vi "Pass Allowed Message.vi"(2 "Allowed Message":string[](array[string]), 3 "JKISM External Event":string) -> (1 "States":string)   [LabVIEW 2017, in "_jkism_magic.lvlib"]
uses:
  _jkism_magic.lvlib
  Communicable State Machine.lvlib
  _Shared/CSM Shared.lvlib
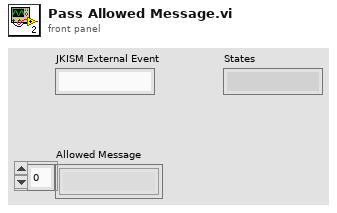
[diagram p1: front panel]
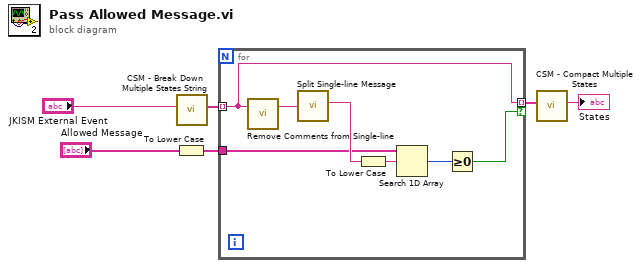
[diagram p0: block diagram]
diagram:
  n1 = To Lower Case(string="Allowed Message") -> (all lower case string=w3:string[])
  n2 = call "CSM - Break Down Multiple States String.vi"("States"="JKISM External Event") -> ("Multiple States"=w1:string[])  [unwired: 10 in]
  n3 = for {
    tunnel: w1 -> [w7] mode=indexing
    tunnel: [w7] -> w4 mode=indexing if=w8
    tunnel: w3 -> [w11]
    n4 = call "Remove Comments from Single-line.vi"("single-line text"=w7) -> ("single-line text without comments"=w13:string)  [unwired: 2 in]
    n5 = call "Split Single-line Message.vi"("single-line text"=w13) -> ("state"=w12:string)  [unwired: 6 in, 3 out]
    n6 = To Lower Case(string=w12) -> (all lower case string=w10:string)
    n7 = Search 1D Array(1D array=w11, element=w10) -> (index of element=w9:i32)  [unwired: 1 in]
    n8 = Greater Or Equal To 0?(x=w9) -> (x >= 0?=w8:bool)
  }
  n9 = call "CSM - Compact Multiple States.vi"("Multiple States"=w4) -> ("States"=→"States":string)  [unwired: 9 in]
